vi "Increase Channel Buffer.vi"(8 "error in (no error)":errorcluster, 9 "Flattened FIFO Config":u8[](array[numeric]), 10 "Channel Index":i32, 11 "CIFCorePlugin in":refnum<class "CIFCorePlugin.lvclass">) -> (0 "error out":errorcluster, 3 "CIFCorePlugin out":refnum<class "CIFCorePlugin.lvclass">)   [LabVIEW 2021, in "CIFCorePlugin.lvclass"]
doc: "This advanced feature will increase the buffer configured for a FIFO channel. It is useful when buffer sizes need to change based on a user configuration.\n\nIt can only be called on the publisher. \nIt will delete the existing buffer and create a new channel with the same name and larger memory buffer. \nThis must be a configuration time change. The channel must not have a linked subscriber and the plugin must be in the listen state. \n\nProvide the channel index to be updated and the new flattened FIFO configuration. Only the size information (bytes per message and number of messages) will be used from the FIFO configuration, all other information will be reused from the existing channel."
uses:
  CIFCorePlugin.lvclass
  CIFCorePlugin.lvclass/CIFCorePlugin.ctl
  <vilib>/CIF Foundation/CIF Channels Core/ChannelCommon/ChannelCommon.lvlib
  Typedef/Energized States.ctl
  Common/CIFCoreCommon.lvlib
  Common/Typedef/Errors.ctl
  <vilib>/CIF Foundation/CIF Channels Core/CIFChannels/CIFChannels.lvclass
  <vilib>/CIF Foundation/CIF Channels Core/CIFChannels/Typedef/Direction.ctl
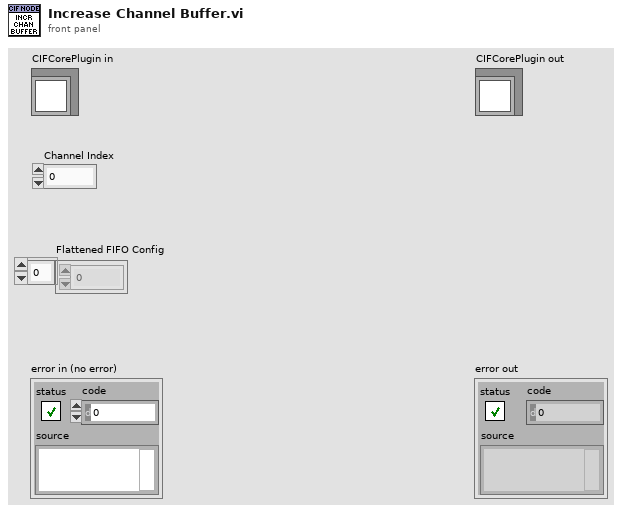
[diagram p1: front panel]
types:
  T1 = typedef "CIFCorePlugin.lvclass/Energized States.ctl" = enum16{"Listen", "Prepare", "Execute", "Housekeep", "Cleanup", "Destroy"}
  T2 = typedef "CIFCoreCommon.lvlib/Errors.ctl" = enum16{"Invalid Clock ID", "Long Sleep", "gRPC Server Not Found", "Config Parse", "Timestamp Wrap", "Delayed Execution", "Duplicate Channel", "Missing Channel", "Incorrect Type", "Flatten Error", "Unflatten Data", "Unique Name", "Plugin Not Found", "Plugin Type Not Found", "Plugin Version Not Found", "Manager Not Found", "Numerical Issue", "Time Jump", "Clock ID Match", "Channel Length", "Plugin Connection", "gRPC Server Connection", "PPL Name Match", "Build", "Config Log Parse", "Plugin Load", "UI Subpanel Load", "Python Name", "Invalid Name", "Unable to Change Ch Buffer"}
  T3 = typedef "CIFChannels.lvclass/Direction.ctl" = enum16{"Publisher", "Subscriber"}
  T4 = typedef "ChannelCommon.lvlib/FIFO Config.ctl" = cluster{"Max Bytes/Msg":u64, "Max Msg/FIFO":u64, "Flags":u64, "Custom Data":u8[]}
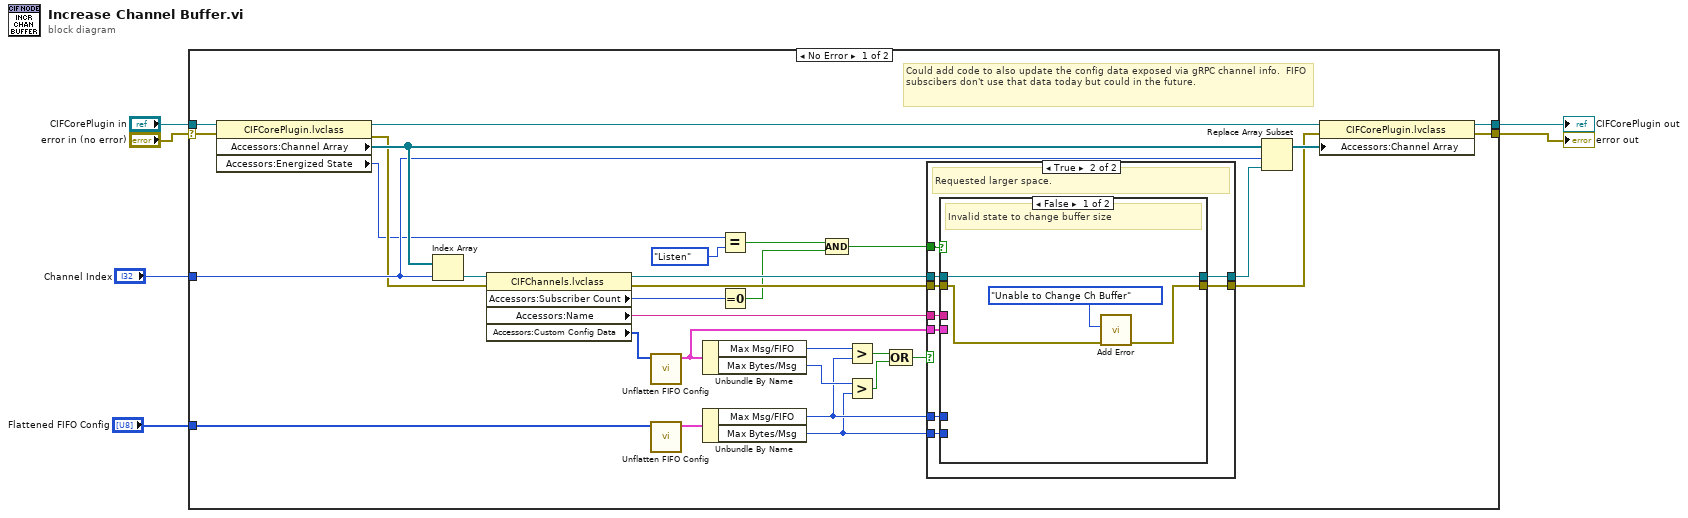
[diagram p0: block diagram]
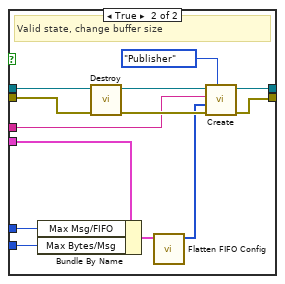
[diagram p3: hidden frame]
diagram:
  n1 = case shown="No Error" "error in (no error)" {
    selector: "error in (no error)" -> [w35 w68]
    tunnel: [w31 w68] -> w5
    tunnel: [w36 w67] -> w3
    tunnel: "CIFCorePlugin in" -> [w38 w67]
    tunnel: "Channel Index" -> [w32 _]
    tunnel: "Flattened FIFO Config" -> [w29 _]
    frame No Error {
      # "Could add code to also update the config data exposed via gRPC channel info.  FIFO subscibers don't use that data today but could in the future."
      n2 = property class="CIFCorePlugin.lvclass"(reference=w38, error in=w35) -> (reference out=w37:refnum<class "CIFCorePlugin.lvclass">, error out=w20:errorcluster, "Accessors:Channel Array"=w34:refnum<class "CIFChannels.lvclass">[], "Accessors:Energized State"=w15:T1)
      n3 = Index Array(array=w34, index=w32) -> (element=w30:refnum<class "CIFChannels.lvclass">)
      n4 = property class="CIFChannels.lvclass"(reference=w30, error in=w20) -> (reference out=w22:refnum<class "CIFChannels.lvclass">, error out=w21:errorcluster, "Accessors:Subscriber Count"=w19:u32, "Accessors:Name"=w9:string, "Accessors:Custom Config Data"=w10:u8[])
      n5 = call <vilib>:"Unflatten FIFO Config.vi"("Flattened Data in"=w10) -> ("FIFO Config out"=w11:T4)  [unwired: 9 in, 1 out]
      n6 = call <vilib>:"Unflatten FIFO Config.vi"("Flattened Data in"=w29) -> ("FIFO Config out"=w28:T4)  [unwired: 9 in, 1 out]
      n7 = Unbundle By Name(w11) -> ("Max Msg/FIFO"=w27:u64, "Max Bytes/Msg"=w26:u64)
      n8 = Unbundle By Name(w28) -> ("Max Msg/FIFO"=w13:u64, "Max Bytes/Msg"=w12:u64)
      n9 = Equal?(x=w15, y=Energized_States."Listen") -> (x = y?=w17:bool)
      n10 = Equal To 0?(x=w19) -> (x = 0?=w18:bool)
      n11 = Compound Arithmetic op=AND(w17, w18) -> (w16:bool)
      n12 = Greater?(x=w27, y=w13) -> (0:w25:bool)
      n13 = Greater?(x=w26, y=w12) -> (0:w24:bool)
      n14 = Compound Arithmetic op=OR(w25, w24) -> (w23:bool)
      n15 = case shown="True" w23 {
        tunnel: w22 -> [w39 w48]
        tunnel: w21 -> [w40 w47]
        tunnel: w16 -> [_ w49]
        tunnel: w13 -> [_ w46]
        tunnel: w12 -> [_ w45]
        tunnel: w11 -> [_ w44]
        tunnel: w9 -> [_ w43]
        tunnel: [w39 w42] -> w8
        tunnel: [w40 w41] -> w7
        frame False {
          # "Requested space is not larger.  No change needed."
        }
        frame True {
          # "Requested larger space."
          n16 = case shown="False" w49 {
            tunnel: w48 -> [w51 w62]
            tunnel: w47 -> [w53 w61]
            tunnel: w46 -> [_ w59]
            tunnel: w45 -> [_ w57]
            tunnel: w44 -> [_ w66]
            tunnel: w43 -> [_ w60]
            tunnel: [w51 w55] -> w42
            tunnel: [w50 w54] -> w41
            frame False {
              # "Invalid state to change buffer size"
              n17 = call "Add Error.vi"("error in (no error)"=w53, "Error"=Errors."Unable to Change Ch Buffer") -> ("error out"=w50:errorcluster)  [unwired: 9 in]
            }
            frame True {
              # "Valid state, change buffer size"
              n18 = Bundle By Name(cluster=w66, "Max Msg/FIFO"=w59, "Max Bytes/Msg"=w57) -> (w58:T4)
              n19 = call-dynamic "Destroy.vi"("error in (no error)"=w61, "CIFChannels in"=w62) -> ("error out"=w63:errorcluster, "CIFChannels out"=w65:refnum<class "CIFChannels.lvclass">)  [unwired: 8 in]
              n20 = call <vilib>:"Flatten FIFO Config.vi"("FIFO Config in"=w58) -> ("Flattened FIFO Config"=w56:u8[])  [unwired: 10 in]
              n21 = call-dynamic "Create.vi"("Direction"=Direction."Publisher", "error in (no error)"=w63, "Custom Config Data"=w56, "Name"=w60, "CIFChannels in"=w65) -> ("error out"=w54:errorcluster, "CIFChannels out"=w55:refnum<class "CIFChannels.lvclass">)  [unwired: 5 in]
            }
          }
        }
      }
      n22 = Replace Array Subset(array=w34, new element=w8, index=w32) -> (w33:refnum<class "CIFChannels.lvclass">[])
      n23 = property class="CIFCorePlugin.lvclass"(reference=w37, error in=w7, "Accessors:Channel Array"=w33) -> (reference out=w36:refnum<class "CIFCorePlugin.lvclass">, error out=w31:errorcluster)
    }
    frame Error {
    }
  }
  "error out" <- w5
  "CIFCorePlugin out" <- w3
